vi "Fake Serial Instrument.vi"() -> ()   [LabVIEW 2020]
uses:
  <vilib>/Instr/_visa.llb/VISA Configure Serial Port (Instr).vi
panel:
  out "Numeric":i32
  in  "stop":bool
  in  "VISA resource name":refnum<visa-resource-name>
  out "error out":errorcluster
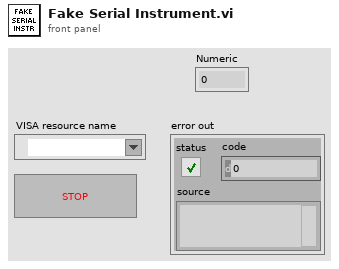
[diagram p1: front panel]
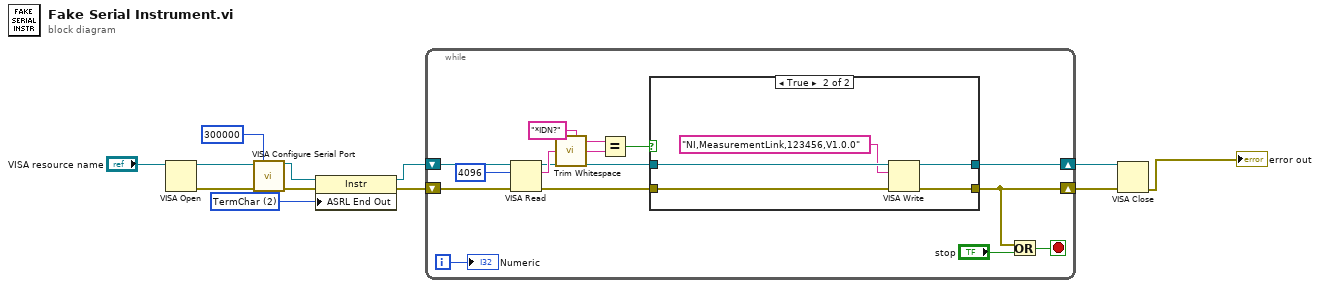
[diagram p0: block diagram]
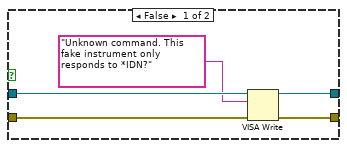
[diagram p2: hidden frame]
diagram:
  w1 = u16 2 items=["None", "Last Bit", "TermChar", "Break"] ("Serial Settings:End Mode for Writes")
  n1 = VISA Open(VISA resource name="VISA resource name") -> (VISA resource name=w7:refnum<visa-resource-name>, error out=w8:errorcluster)  [unwired: 4 in]
  n2 = call-poly "VISA Configure Serial Port"("VISA resource name"=w7, "timeout (10sec)"=u32 300000, "error in (no error)"=w8) -> ("VISA resource name out"=w3:refnum<visa-resource-name>, "error out"=w5:errorcluster)  [unwired: 11 in]
  n3 = property class="Instr"(reference=w3, error in=w5, "ASRL End Out"=w1) -> (reference out=w2:refnum<visa-resource-name>, error out=w4:errorcluster)
  n4 = while {
    shift-right: [w16] -> w10
    shift-left: w2 -> [w25]
    shift-right: [w15] -> w11
    shift-left: w4 -> [w24]
    i -> [w14]
    stop <- w23 stop-if-true
    n5 = VISA Read(VISA resource name=w25, byte count=u32 4096, error in (no error)=w24) -> (VISA resource name out=w17:refnum<visa-resource-name>, read buffer=w21:string, error out=w18:errorcluster)  [unwired: 1 out]
    n6 = call <vilib>:"Trim Whitespace.vi"("string"=w21) -> ("trimmed string"=w13:string)  [unwired: 1 in]
    n7 = Equal?(x="*IDN?", y=w13) -> (x = y?=w19:bool)
    n8 = case shown="True" w19 {
      tunnel: w18 -> [w31 w36]
      tunnel: w17 -> [w30 w35]
      tunnel: [w29 w34] -> w16
      tunnel: [w28 w33] -> w15
      frame False {
        n9 = VISA Write(VISA resource name=w30, write buffer="Unknown command. This fake instrument only responds to *IDN?", error in (no error)=w31) -> (VISA resource name out=w29:refnum<visa-resource-name>, error out=w28:errorcluster)  [unwired: 1 out]
      }
      frame True {
        n10 = VISA Write(VISA resource name=w35, write buffer="NI,MeasurementLink,123456,V1.0.0", error in (no error)=w36) -> (VISA resource name out=w34:refnum<visa-resource-name>, error out=w33:errorcluster)  [unwired: 1 out]
      }
    }
    n11 = Or(x=w15, y="stop") -> (x .or. y?=w23:bool)
    "Numeric" <- w14
  }
  n12 = VISA Close(VISA resource name=w10, error in (no error)=w11) -> (error out=→"error out":errorcluster)
